vi "TorqueMotorMonitor.vi"   [LabVIEW 2015]
uses:
  Instrument_Setup.vi
  Global/Global Variables/Data_Display_global.vi
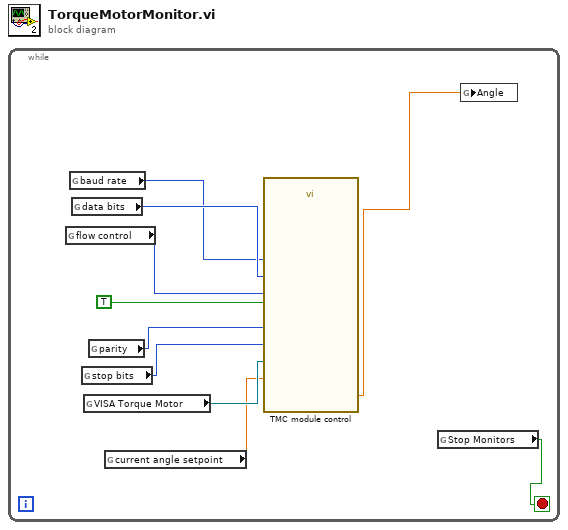
[diagram p0: block diagram]
diagram:
  n1 = while {
    stop <- w1 stop-if-true
    n2 = global read "Instrument_Setup.vi" "flow control"() -> (w10:u16)
    n3 = global read "Instrument_Setup.vi" "baud rate"() -> (w8:u32)
    n4 = global read "Instrument_Setup.vi" "data bits"() -> (w9:u16)
    n5 = global read "Instrument_Setup.vi" "stop bits"() -> (w6:u16)
    n6 = global read "Instrument_Setup.vi" "VISA Torque Motor"() -> (w4:refnum<visa-resource-name>)
    n7 = global read "Instrument_Setup.vi" "parity"() -> (w7:u16)
    n8 = global read "Data_Display_global.vi" "current angle setpoint"() -> (w3:dbl)
    n9 = call "TMC module control.vi"("Nur Position auslesen"=TRUE, "Winkel [°]"=w3, "flow control"=w10, "VISA resource name"=w4, "stop bits"=w6, "parity"=w7, "data bits"=w9, "baud rate"=w8) -> ("Ausgelesener Winkel [°]"=w2:dbl)  [unwired: 1 out]
    n10 = global read "Data_Display_global.vi" "Stop Monitors"() -> (w1:bool)
    n11 = global write "Data_Display_global.vi" "Angle"(w2) -> ()
  }
